vi "Close.vi"(8 "error in":errorcluster, 11 "Flow Gradient in":refnum<class "Flow Gradient.lvclass">) -> (0 "error out":errorcluster, 3 "Flow Gradient out":refnum<class "Flow Gradient.lvclass">)   [LabVIEW 2023, in "Flow Gradient.lvclass"]
uses:
  Flow Gradient.lvclass
  Parents/Gradient/Gradient.lvclass
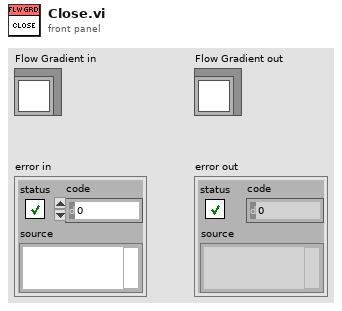
[diagram p1: front panel]
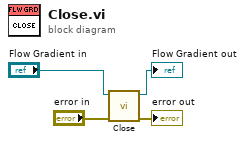
[diagram p0: block diagram]
diagram:
  n1 = call-parent "Close.vi"("error in"="error in", "Gradient in"="Flow Gradient in") -> ("error out"=→"error out":errorcluster, "Gradient out"=→"Flow Gradient out":refnum<class "Flow Gradient.lvclass">)  [unwired: 8 in]
